vi "AdventCode_Main.vi"() -> ()   [LabVIEW 2020]
uses:
  PuzzleBase_class/PuzzleBase.lvclass
  AdventCode_class/AdventCode.lvclass
panel:
  out "Result 2":u64=148962
  out "Result 1":u64=4659
  in  "Day":i32=16 min=1 max=25
  in  "Year":i32=2021 min=2020 max=2021
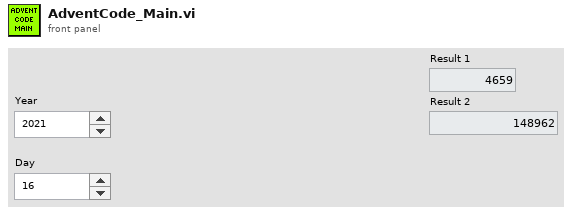
[diagram p1: front panel]
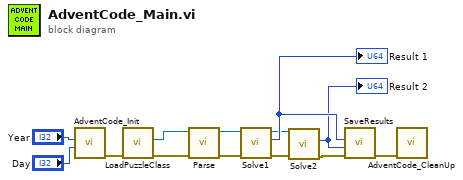
[diagram p0: block diagram]
diagram:
  n1 = call "AdventCode_Init.vi"("Day"="Day", "Year"="Year") -> ("Error Out"=w7:errorcluster)  [unwired: 7 in, 2 out]
  n2 = call "LoadPuzzleClass.vi"("Error In"=w7) -> ("Error Out"=w5:errorcluster, "PuzzleBase"=w6:refnum<class "PuzzleBase.lvclass">)  [unwired: 9 in]
  n3 = call-dynamic "Parse.vi"("Error In"=w5, "reference in"=w6) -> ("Error Out"=w13:errorcluster, "reference out"=w12:refnum<class "PuzzleBase.lvclass">)  [unwired: 8 in]
  n4 = call-dynamic "Solve1.vi"("Error In"=w13, "reference in"=w12) -> ("Error Out"=w3:errorcluster, "Result"=w11:u64, "reference out"=w4:refnum<class "PuzzleBase.lvclass">)  [unwired: 7 in]
  "Result 1" <- w11
  n5 = call-dynamic "Solve2.vi"("Error In"=w3, "reference in"=w4) -> ("Error Out"=w2:errorcluster, "Result"=w1:u64)  [unwired: 7 in, 1 out]
  "Result 2" <- w1
  n6 = call "SaveResults.vi"("Error In"=w2, 9:"Result 2"=w1, 10:"Result 2"=w11) -> ("Error Out"=w10:errorcluster)  [unwired: 8 in]
  n7 = call "AdventCode_CleanUp.vi"("Error In"=w10) -> ()  [unwired: 10 in, 1 out]
